vi "Get Address.vi"(8 "Error in":errorcluster, 11 "7 - Bit Addressing in":refnum<class "7 - Bit Addressing.lvclass">) -> (0 "Error out":errorcluster, 3 "7 - Bit Addressing out":refnum<class "7 - Bit Addressing.lvclass">)   [LabVIEW 2020, in "7 - Bit Addressing.lvclass"]
uses:
  7 - Bit Addressing.lvclass
  C:/LV Assignments/SDLC VI/Class/Parent Class/Address/Address.lvclass
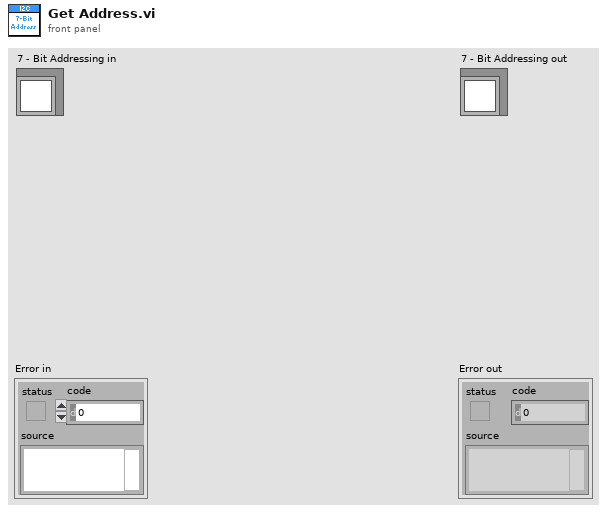
[diagram p1: front panel]
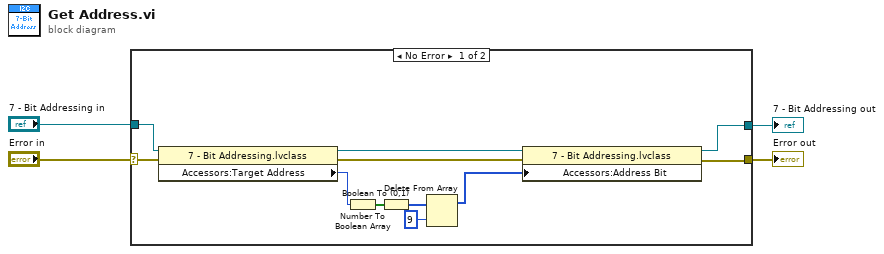
[diagram p0: block diagram]
diagram:
  n1 = case shown="No Error" "Error in" {
    selector: "Error in" -> [w14 w17]
    tunnel: [w7 w17] -> w3
    tunnel: [w6 w16] -> w1
    tunnel: "7 - Bit Addressing in" -> [w15 w16]
    frame No Error {
      n2 = property class="7 - Bit Addressing.lvclass"(reference=w15, error in=w14) -> (reference out=w9:refnum<class "7 - Bit Addressing.lvclass">, error out=w8:errorcluster, "Accessors:Target Address"=w13:i16)
      n3 = Number To Boolean Array(number=w13) -> (Boolean array=w12:bool[])
      n4 = Boolean To (0,1)(Boolean=w12) -> (0, 1=w11:i16[])
      n5 = Delete From Array(array=w11, length=9) -> (array with subset deleted=w5:i16[])  [unwired: 1 in, 1 out]
      n6 = property class="7 - Bit Addressing.lvclass"(reference=w9, error in=w8, "Accessors:Address Bit"=w5) -> (reference out=w6:refnum<class "7 - Bit Addressing.lvclass">, error out=w7:errorcluster)
    }
    frame Error {
    }
  }
  "Error out" <- w3
  "7 - Bit Addressing out" <- w1
